vi "Start.vi"(6 "Self Alias":string, 8 "Actor":refnum<class "Actor.lvclass">, 9 "Creator Attributes":T1, 10 "Queue of Created Init":refnum<queue>) -> (0 "error out":errorcluster)   [LabVIEW 2020, in "jettl.lvlib" / "Actor.lvlib" / "Base Actor.lvclass"]
uses:
  Base Actor.lvclass
  Actor/Actor.lvclass
  Msg/Msg.lvclass
  Actor.vi
  Implemented Msgs.ctl
  Actor.lvlib
  Attributes.ctl
  Created Init.ctl
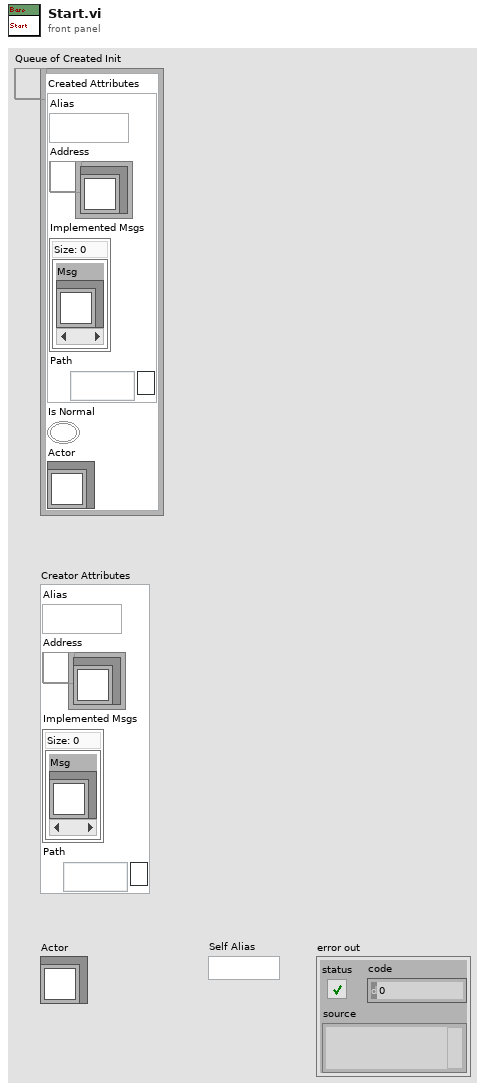
[diagram p1: front panel]
types:
  T1 = typedef "jettl.lvlib/Actor.lvlib/Attributes.ctl" = cluster{"Alias":string, "Address":refnum<user-event>, "Implemented Msgs":T2, "Path":path}
  T2 = typedef "jettl.lvlib/Actor.lvlib/Implemented Msgs.ctl" = set{refnum<class "Msg.lvclass">}
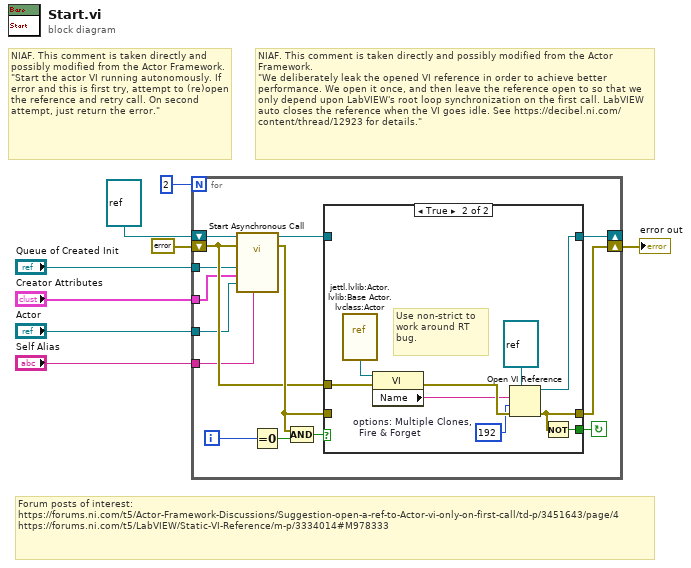
[diagram p0: block diagram]
diagram:
  # "Forum posts of interest:\nhttps://forums.ni.com/t5/Actor-Framework-Discussions/Suggestion-open-a-ref-to-Actor-vi-only-on-first-call/td-p/3451643/page/4\nhttps://forums.ni.com/t5/LabVIEW/Static-VI-Reference/m-p/3334014#M978333"
  # "NIAF. This comment is taken directly and possibly modified from the Actor Framework.\n\"We deliberately leak the opened VI reference in order to achieve better performance. We open it once, and then leave the reference open to so that we only depend upon LabVIEW's root loop synchronization on the first call. LabVIEW auto closes the reference when the VI goes idle. See https://decibel.ni.com/content/thread/12923 for details.\""
  # "NIAF. This comment is taken directly and possibly modified from the Actor Framework.\n\"Start the actor VI running autonomously. If error and this is first try, attempt to (re)open the reference and retry call. On second attempt, just return the error.\""
  n1 = for {
    N: 2 -> [_]
    shift-right: [w22] -> _
    shift-left: refnum<vi> refnum -> [w21]
    shift-right: [w19] -> w6
    shift-left: errorcluster {"status"=FALSE, "code"=0, "source"=""} ("error out") -> [w13]
    tunnel: "Queue of Created Init" -> [w10]
    tunnel: "Actor" -> [w11]
    tunnel: "Self Alias" -> [w12]
    tunnel: "Creator Attributes" -> [w9]
    i -> [w16]
    stop <- w14 continue-if-true
    n2 = call-by-ref "Start Asynchronous Call"(reference=w21, error in=w13, "Self Alias"=w12, "Actor"=w11, "Creator Attributes"=w9, "Queue of Created Init"=w10) -> (reference out=w20:refnum<vi>, error out=w15:errorcluster)  [unwired: 8 in]
    n3 = Equal To 0?(x=w16) -> (x = 0?=w17:bool)
    n4 = Compound Arithmetic op=AND(w15, w17) -> (w18:bool)
    n5 = case shown="True" w18 {
      tunnel: [w24 w30] -> w22
      tunnel: [w23 w28] -> w19
      tunnel: w20 -> [w24 _]
      tunnel: w15 -> [w23 _]
      tunnel: [_ w29] -> w14
      tunnel: w13 -> [_ w27]
      frame False {
      }
      frame True {
        w31 = 192  # options: Multiple Clones,   Fire & Forget
        # "Use non-strict to work around RT bug."
        n6 = vi-ref "jettl.lvlib:Actor.lvlib:Base Actor.lvclass:Actor.vi"() -> (w26:refnum<vi>)
        n7 = property class="VI"(reference=w26, error in=w27) -> (error out=w33:errorcluster, "Name"=w32:string)  [unwired: 1 out]
        n8 = Open VI Reference(type specifier VI Refnum (for type only)=refnum<vi> refnum, vi path=w32, options=w31, error in (no error)=w33) -> (vi reference=w30:refnum<vi>, error out=w28:errorcluster)  [unwired: 2 in]
        n9 = Not(x=w28) -> (.not. x?=w29:bool)
      }
    }
  }
  "error out" <- w6
